vi "Get Identifier.vi"(8 "error in (no error)":errorcluster, 11 "NI-XNET CAN Reader Execution Unit in":refnum<class "NI-XNET CAN Reader Execution Unit.lvclass">) -> (0 "error out":errorcluster, 2 "Identifier":string, 3 "NI-XNET CAN Reader Execution Unit out":refnum<class "NI-XNET CAN Reader Execution Unit.lvclass">)   [LabVIEW 2020, in "Communication Bus Template Engine.lvlib" / "Implementation.lvlib" / "NI-XNET CAN Reader Execution Unit.lvclass"]
uses:
  NI-XNET CAN Reader Execution Unit.lvclass
  NI-XNET CAN Reader Execution Unit.lvclass/NI-XNET CAN Reader Execution Unit.ctl
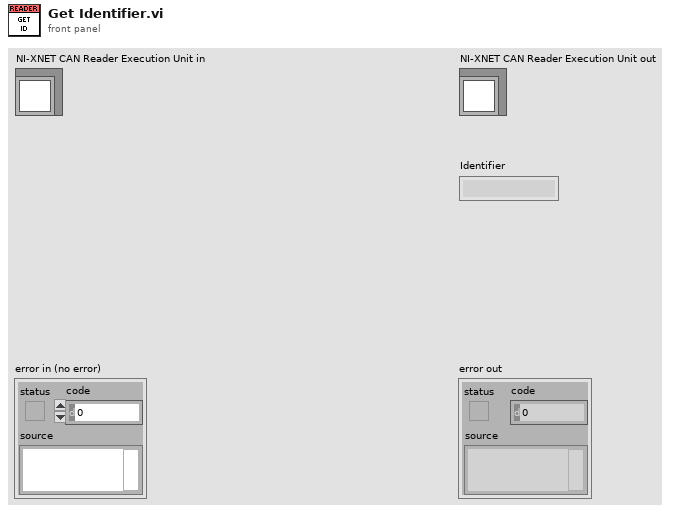
[diagram p1: front panel]
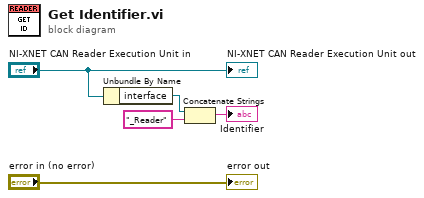
[diagram p0: block diagram]
diagram:
  n1 = Unbundle By Name("NI-XNET CAN Reader Execution Unit in") -> ("interface"=w5:refnum<k21>)
  n2 = Concatenate Strings(w5, "_Reader" ("string")) -> (→"Identifier":string)
  "error out" <- "error in (no error)"
  "NI-XNET CAN Reader Execution Unit out" <- "NI-XNET CAN Reader Execution Unit in"
